vi "gyro pll async.vi"(11 "pll event pair":T8) -> ()   [LabVIEW 2018]
uses:
  agregator -- action.ctl
  four-corner circle transformation.ctl
  interpolation state - real.ctl
  PID action.ctl
  data source action.ctl
  publisher action.ctl
  pll talkback data type.ctl
  server talkback message type.ctl
  pid -- parameters.ctl
  PID - mode.ctl
  pll parameters.ctl
  lorentzian.ctl
  circle corners.ctl
  server talkto message type.ctl
  server talk-to-back pair.ctl
panel:
  in  "main":enum32{"Page 1", "Page 2", "Page 3"}(tab)
  in  "pll parameters":T1={"PID mode"=enum."normal", "plot hist time (sec)"=1.0, "dt (sec)"=0.001, "visc hist time (sec)"=2.0, "time int ave time (sec)"=0.3, "PLL limits (Hz)"=5000.0} {"PLL limits (Hz)" format="%#.2f"; "time int ave time (sec)" format="%#_10f"; "visc hist time (sec)" format="%#_10f"; "dt (sec)" format="%#_10f"; "plot hist time (sec)" format="%#_10f"}
  in  "PID parameters :{}[];'":T3={"I (sec)"=0.004634123928756344, "P (sec)"=0.008980860327047186} {"P (sec)" scale=0.01..10.0; "I (sec)" scale=0.01..10.0}
  out "results":T4={"freq (Hz)"=40017.438097734725, "gamma (Hz)"=6.817921124952451, "Voltage (V)"=6.817921124952451+0.0i, "overlimit ?"=FALSE} {"Voltage (V)" format="%#.4f"; "gamma (Hz)" format="%#.4f"; "freq (Hz)" format="%#.11f"}
  out "PLL is ON ?":bool
  in  "Do reset frequency -- PID action":T5=enum."reset frequency"
  in  "Do reset frequency source":dbl=15.0 format="%#_10f"
  out "zi freq temporary":dbl=40015.59220124337 format="%#.2f"
  out "DO reset freq !":bool
  in  "lorentzian":T6={"A (VHz)"=1.0, "f (Hz)"=1000.0, "G (Hz)"=3.0, "phi(rad)"=0.0, "Q"=300.0, "Norm  Ampl"=nan, "bg (V)"=0.0+0.0i, "4corners"={"z (-pi/2)"=9.277908004825974e-07+0.0007240755403629966i, "z(inf)"=2.6527949823343002e-05+0.0007477540585896028i, "z (pi/2)"=2.8494315967368497e-06+0.0007733542176124632i, "z center"=1.8886111986097237e-06+0.0007487148789877299i, "z(0)"=-2.2750727426123552e-05+0.000749675699385857i, "radius"=2.4658065287076567e-05}} {"bg (V)" format="%#9_9f"; "Q" format="%#9_9f"; "phi(rad)" format="%#9_9f"; "G (Hz)" format="%#9_9f"; "f (Hz)" format="%#9_9f"}
  out "Stoped?":bool
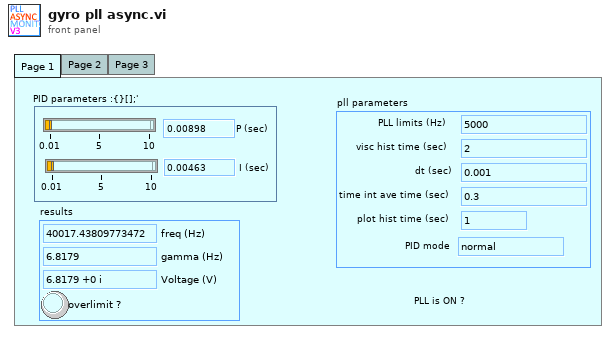
[diagram p1: front panel]
types:
  T1 = typedef "pll parameters.ctl" = cluster{"PID mode":T2, "plot hist time (sec)":dbl, "dt (sec)":dbl, "visc hist time (sec)":dbl, "time int ave time (sec)":dbl, "PLL limits (Hz)":dbl}
  T2 = typedef "PID - mode.ctl" = enum16{"normal", "heat"}
  T3 = typedef "pid -- parameters.ctl" = cluster{"I (sec)":dbl, "P (sec)":dbl}
  T4 = typedef "pll talkback data type.ctl" = cluster{"freq (Hz)":dbl, "gamma (Hz)":dbl, "Voltage (V)":cdb, "overlimit ?":bool}
  T5 = typedef "PID action.ctl" = enum16{"append", "empty!", "reset frequency", "reset from num", "overlimit"}
  T6 = typedef "lorentzian.ctl" = cluster{"A (VHz)":dbl, "f (Hz)":dbl, "G (Hz)":dbl, "phi(rad)":dbl, "Q":dbl, "Norm  Ampl":dbl, "bg (V)":cdb, "4corners":T7}
  T7 = typedef "circle corners.ctl" = cluster{"z (-pi/2)":cdb, "z(inf)":cdb, "z (pi/2)":cdb, "z center":cdb, "z(0)":cdb, "radius":dbl}
  T8 = typedef "server talk-to-back pair.ctl" = cluster{"talkback event":refnum<user-event>, "talkto event":refnum<user-event>}
  T9 = typedef "interpolation state - real.ctl" = cluster{"requested size":i32, "Array":dbl[], "actual number of elements":i32}
  T10 = typedef "agregator -- action.ctl" = enum16{"append", "interpolate", "empty!", "force", "init", "scale", "read last"}
  T11 = typedef "server talkback message type.ctl" = cluster{"message":enum16{"new", "void"}}
  T12 = typedef "publisher action.ctl" = enum16{"set", "get", "init", "check"}
  T13 = typedef "data source action.ctl" = enum16{"set", "get", "init", "set-and-get", "init source"}
  T14 = typedef "four-corner circle transformation.ctl" = enum16{"z(c) z(inf)", "z(c) z(zero)", "fix phase", "calculate lorentzian", "z(0) z(+-pi/2)", "shift to zcenter", "to  canonical", "get canonical phase", "get4corners", "update lorentzian -- from z0", "fake gamma normal", "fake gamma heat", "calculate complex slope"}
  T15 = typedef "PLL data source.ctl" = enum16{"meta", "MFLI", "SRS865A", "arydh"}
  T16 = typedef "interpolation state - complex.ctl" = cluster{"requested size":i32, "Array":cdb[], "actual number of elements":i32}
  T17 = enum16{"stop", "start", "update pars", "update request", "new", "launch", "exit", "get", "reset", "pause", "unpause"}
  T18 = typedef "eventvkey.ctl" = enum16{"ASCII", "Enter", "Return", "Shift", "Ctrl", "Alt", "Cmd", "Opt", "Caps", "NumLock", "Clear", "Break", "Up", "Down", "Left", "Right", "Insert", "Delete", "Home", "End", "PageUp", "PageDown", "Escape", "Help", "Pause", "ScrollLock", "F1", "F2", "F3", "F4", "F5", "F6", "F7", "F8", "F9", "F10", "F11", "F12", "F13", "F14", "F15", "F16", "F17", "F18", "F19", "F20", "F21", "F22", "F23", "F24", "Play", "VolumeUp", "VolumeDown", "Mute", "Two Byte Char"}
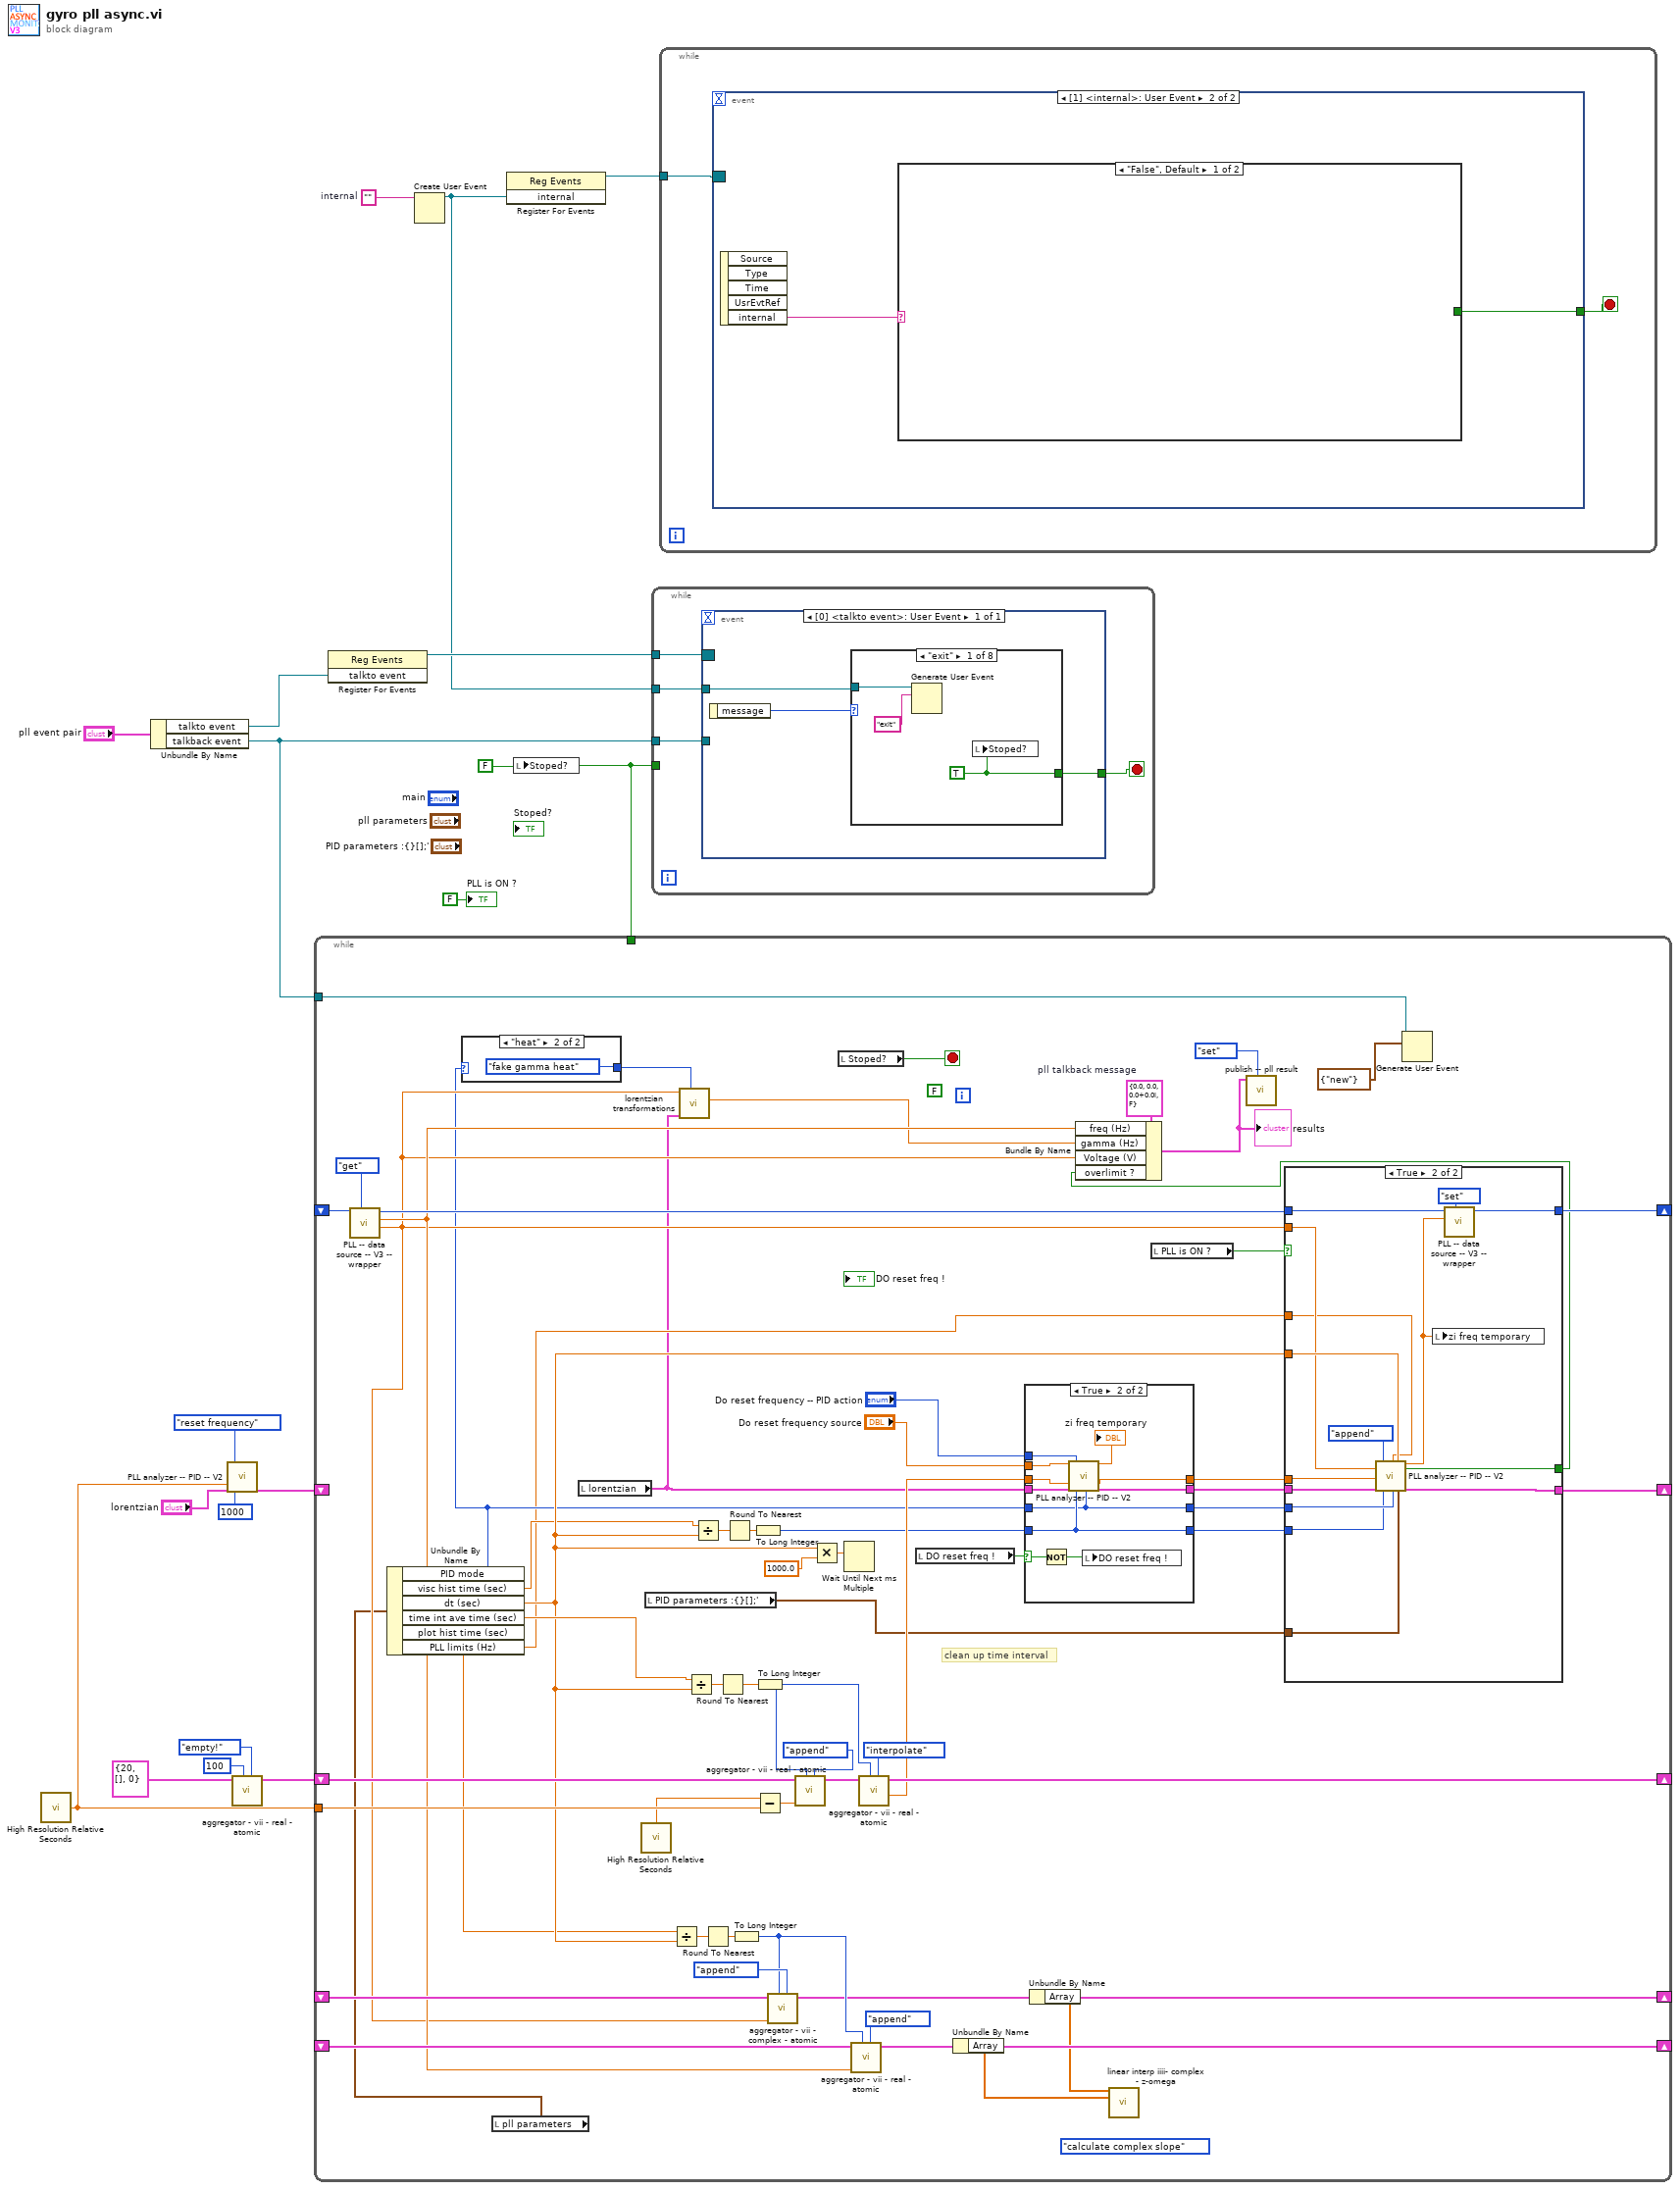
[diagram p0: block diagram]
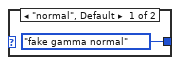
[diagram p2: hidden frame]
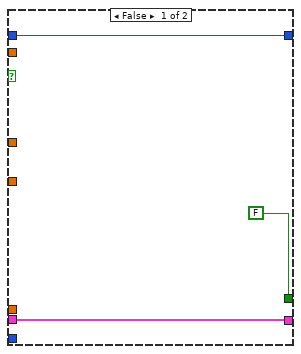
[diagram p3: hidden frame]
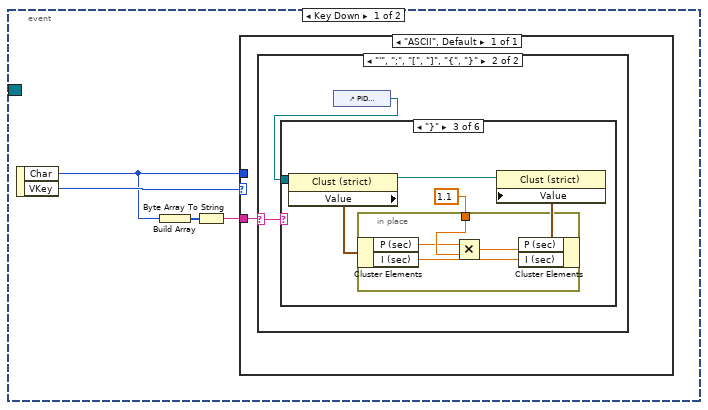
[diagram p5: hidden frame]
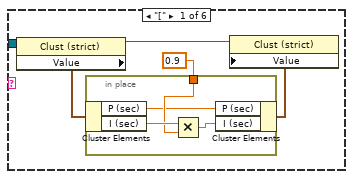
[diagram p7: hidden frame]
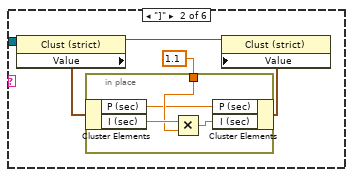
[diagram p8: hidden frame]
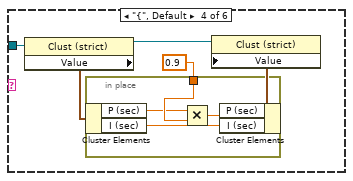
[diagram p9: hidden frame]
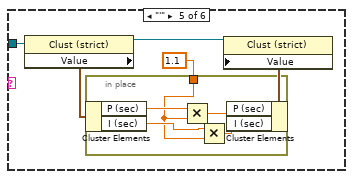
[diagram p10: hidden frame]
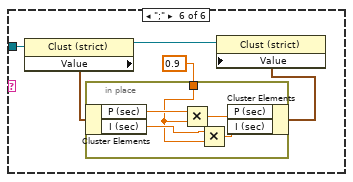
[diagram p11: hidden frame]
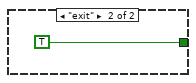
[diagram p12: hidden frame]
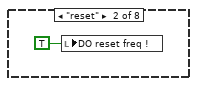
[diagram p13: hidden frame]
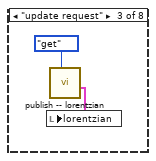
[diagram p14: hidden frame]
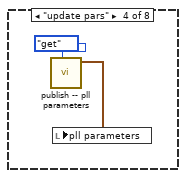
[diagram p15: hidden frame]
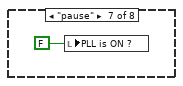
[diagram p18: hidden frame]
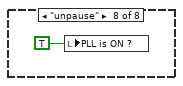
[diagram p19: hidden frame]
diagram:
  w3 = ""  # internal
  w4 = FALSE ("Stop")
  n1 = call <vilib>:"High Resolution Relative Seconds.vi"() -> ("relative seconds"=w6:dbl)
  n2 = Unbundle By Name("pll event pair") -> ("talkto event"=w14:refnum<user-event>, "talkback event"=w15:refnum<user-event>)
  n3 = call "PLL analyzer -- PID -- V2.vi"("time in (sec)"=w6, "lorentzian IN"="lorentzian", "PID action"=PID_action."reset frequency", "requested size"=1000) -> ("lorentzian  OUT"=w9:T6)  [unwired: 12 in, 3 out]
  n4 = call "aggregator - vii - real - atomic.vi"("aggregator action"=agregator_--_action."empty!", "requested size"=100, "state IN"=T9 {"requested size"=20, "Array"=[], "actual number of elements"=0}) -> ("state OUT"=w12:T9)  [unwired: 5 in, 3 out]
  n5 = while {
    tunnel: w6 -> [w79]
    shift-right: [w77] -> _
    shift-left: w9 -> [_]
    shift-right: [w43] -> _
    shift-left: _ -> [w76]
    shift-right: [w72] -> _
    shift-left: _ -> [w73]
    shift-right: [w67] -> _
    shift-left: w12 -> [w70]
    shift-right: [w62] -> _
    shift-left: _ -> [w58]
    tunnel: w15 -> [w20]
    tunnel: w4 -> [_]
    stop <- w23 stop-if-true
    (unwired) FALSE
    w35 = T4 {"freq (Hz)"=0.0, "gamma (Hz)"=0.0, "Voltage (V)"=0.0+0.0i, "overlimit ?"=FALSE}  # pll talkback message
    (unwired) four-corner_circle_transformation."calculate complex slope" ("4 corner circle transformation")
    # "clean up time interval"
    n6 = call "PLL -- data source -- V3 -- wrapper.vi"("data source action"=data_source_action."get", "PLL data source"=w58) -> ("z out (V)"=w38:cdb, "Freq out (Hz)"=w42:dbl, "PLL data source OUT"=w60:T15)  [unwired: 7 in]
    n7 = local read "pll parameters"() -> (w30:T1)
    n8 = Unbundle By Name(w30) -> ("PID mode"=w31:T2, "visc hist time (sec)"=w32:dbl, "dt (sec)"=w33:dbl, "time int ave time (sec)"=w34:dbl, "plot hist time (sec)"=w29:dbl, "PLL limits (Hz)"=w27:dbl)
    n9 = case shown="\"heat\"" w31 {
      tunnel: [four-corner_circle_transformation."fake gamma normal" ("4 corner circle transformation") four-corner_circle_transformation."fake gamma heat" ("4 corner circle transformation")] -> w40
      frame "normal", Default {
      }
      frame "heat" {
      }
    }
    n10 = local read "lorentzian"() -> (w24:T6)
    n11 = call <vilib>:"High Resolution Relative Seconds.vi"() -> ("relative seconds"=w61:dbl)
    n12 = local read "PID parameters :{}[];'"() -> (w21:T3)
    n13 = Divide(x=w29, y=w33) -> (x/y=w47:dbl)
    n14 = call "lorentzian transformations.vi"("4 corner circle transformation"=w40, "lorentzian in"=w24, "voltage in"=w38) -> ("gamma OUT"=w39:dbl)  [unwired: 5 in, 3 out]
    n15 = Divide(x=w34, y=w33) -> (x/y=w51:dbl)
    n16 = Divide(x=w32, y=w33) -> (x/y=w54:dbl)
    n17 = Round To Nearest(number=w47) -> (nearest integer value=w46:dbl)
    n18 = Round To Nearest(number=w51) -> (nearest integer value=w50:dbl)
    n19 = Round To Nearest(number=w54) -> (nearest integer value=w53:dbl)
    n20 = To Long Integer(number=w46) -> (32bit integer=w45:i32)
    n21 = To Long Integer(number=w53) -> (32bit integer=w52:i32)
    n22 = To Long Integer(number=w50) -> (32bit integer=w49:i32)
    n23 = Subtract(x=w61, y=w79) -> (x-y=w69:dbl)
    n24 = call "aggregator - vii - complex - atomic.vi"("aggregator action"=agregator_--_action."append", "requested size"=w45, "number"=w38, "state IN"=w76) -> ("state OUT"=w43:T16)  [unwired: 4 in, 3 out]
    n25 = call "aggregator - vii - real - atomic.vi"("aggregator action"=agregator_--_action."append", "requested size"=w49, "number"=w69, "state IN"=w70) -> ("state OUT"=w68:T9)  [unwired: 4 in, 3 out]
    n26 = Multiply(x=w33, y=1000.0) -> (x*y=w65:dbl)
    n27 = local read "Stoped?"() -> (w23:bool)
    n28 = Wait Until Next ms Multiple(millisecond multiple=w65) -> ()  [unwired: 1 out]
    n29 = call "aggregator - vii - real - atomic.vi"("aggregator action"=agregator_--_action."append", "requested size"=w45, "number"=w42, "state IN"=w73) -> ("state OUT"=w72:T9)  [unwired: 4 in, 3 out]
    n30 = call "aggregator - vii - real - atomic.vi"("aggregator action"=agregator_--_action."interpolate", "requested size"=w49, "state IN"=w68) -> ("interp average"=w56:dbl, "state OUT"=w67:T9)  [unwired: 5 in, 2 out]
    n31 = local read "DO reset freq !"() -> (w64:bool)
    n32 = Unbundle By Name(w72) -> ("Array"=w36:dbl[])
    n33 = case shown="True" w64 {
      selector: w64 -> [_ w112]
      tunnel: w24 -> [w103 w114]
      tunnel: [w103 w113] -> w63
      tunnel: w52 -> [w102 w109]
      tunnel: [w102 w109] -> w57
      tunnel: w56 -> [w101 w108]
      tunnel: "Do reset frequency -- PID action" -> [_ w107]
      tunnel: "Do reset frequency source" -> [_ w106]
      tunnel: [w101 w105] -> w48
      tunnel: w31 -> [w100 w104]
      tunnel: [w100 w104] -> w44
      frame False {
      }
      frame True {
        n34 = Not(x=w112) -> (.not. x?=w111:bool)
        n35 = call "PLL analyzer -- PID -- V2.vi"("frequency IN (Hz)"=w106, "time in (sec)"=w108, "lorentzian IN"=w114, "PID action"=w107, "requested size"=w109, "PID mode"=w104) -> ("frequency OUT (Hz)"=→"zi freq temporary":dbl, "time out (sec)"=w105:dbl, "lorentzian  OUT"=w113:T6)  [unwired: 10 in, 1 out]
        n36 = local write "DO reset freq !"(w111) -> ()
      }
    }
    n37 = Unbundle By Name(w43) -> ("Array"=w37:cdb[])
    n38 = call "linear interp iiii- complex - z-omega.vi"("z"=w37, "omega"=w36) -> ()  [unwired: 5 in, 9 out]
    n39 = local read "PLL is ON ?"() -> (w22:bool)
    n40 = case shown="True" w22 {
      tunnel: [w84 w99] -> w77
      tunnel: w57 -> [_ w90]
      tunnel: w38 -> [_ w88]
      tunnel: w48 -> [_ w94]
      tunnel: w63 -> [w84 w91]
      tunnel: [w83 w97] -> w62
      tunnel: w60 -> [w83 w95]
      tunnel: w33 -> [_ w93]
      tunnel: w44 -> [_ w92]
      tunnel: w21 -> [_ w87]
      tunnel: [FALSE w86] -> w28
      tunnel: w27 -> [_ w85]
      frame False {
      }
      frame True {
        n41 = call "PLL analyzer -- PID -- V2.vi"("voltage IN (V)"=w88, "time in (sec)"=w94, "lorentzian IN"=w91, "PID action"=PID_action."append", "requested size"=w90, "PLL limits (Hz)"=w85, "PID mode"=w92, "dt (sec)"=w93, "PID parameters"=w87) -> ("frequency OUT (Hz)"=w89:dbl, "overlimit ?"=w86:bool, "lorentzian  OUT"=w99:T6)  [unwired: 7 in, 1 out]
        n42 = local write "zi freq temporary"(w89) -> ()
        n43 = call "PLL -- data source -- V3 -- wrapper.vi"("data source action"=data_source_action."set", "Freq in (Hz)"=w89, "PLL data source"=w95) -> ("PLL data source OUT"=w97:T15)  [unwired: 6 in, 2 out]
      }
    }
    n44 = Bundle By Name(cluster=w35, "freq (Hz)"=w42, "gamma (Hz)"=w39, "Voltage (V)"=w38, "overlimit ?"=w28) -> (w26:T4)
    "results" <- w26
    n45 = call "publish -- pll result.vi"("publisher action"=publisher_action."set", "pll result IN"=w26) -> ()  [unwired: 9 in, 1 out]
    n46 = Generate User Event(user event=w20, event data cluster=T11 {"message"=enum."new"} ("event data")) -> ()  [unwired: 2 in, 2 out]
  }
  n47 = register-events(w14) -> (reference out=w18:refnum<event-registration>)  [unwired: 2 in, 1 out]
  n48 = Create User Event(user event datatype=w3) -> (user event=w1:refnum<user-event>)  [unwired: 1 in, 1 out]
  n49 = register-events(w1) -> (reference out=w2:refnum<event-registration>)  [unwired: 2 in, 1 out]
  n50 = local write "Stoped?"(w4) -> ()
  n51 = while {
    tunnel: w18 -> [w118]
    tunnel: w15 -> [w117]
    tunnel: w4 -> [_]
    tunnel: w1 -> [w115]
    stop <- w116 stop-if-true
    n52 = event shown="[0] <talkto event>: User Event" {
      selector: w118 -> [_]
      dyn-events: _ -> [_]
      timeout: _ -> [_]
      tunnel: w117 -> [_]
      tunnel: [w120] -> w116
      tunnel: w115 -> [w119]
      event User Event {
        n53 = event-data() -> ("message"=w121:T17)  [unwired: 1 in]
        n54 = case shown="\"exit\"" w121 {
          tunnel: [w124 _ _ _ _ _ _ _] -> w120
          tunnel: w119 -> [w123 _ _ _ _ _ _ _]
          frame "exit" {
            w124 = TRUE
            n55 = Generate User Event(user event=w123, event data cluster="exit" ("event data")) -> ()  [unwired: 2 in, 2 out]
            n56 = local write "Stoped?"(w124) -> ()
          }
          frame "reset" {
            n57 = local write "DO reset freq !"(TRUE) -> ()
          }
          frame "update request" {
            n58 = call "publish -- lorentzian.vi"("publisher action"=publisher_action."get") -> ("lorentzian OUT"=w126:T6)  [unwired: 10 in]
            n59 = local write "lorentzian"(w126) -> ()
          }
          frame "update pars" {
            n60 = call "publish -- pll parameters.vi"("publisher action"=publisher_action."get") -> ("pll parameters OUT"=w128:T1)  [unwired: 10 in]
            n61 = local write "pll parameters"(w128) -> ()
          }
          frame "start", Default {
          }
          frame "stop" {
          }
          frame "pause" {
            n62 = local write "PLL is ON ?"(FALSE ("Stoped?")) -> ()
          }
          frame "unpause" {
            n63 = local write "PLL is ON ?"(TRUE ("Stoped?")) -> ()
          }
        }
      }
    }
  }
  n64 = while {
    tunnel: w2 -> [w133]
    stop <- w132 stop-if-true
    n65 = event shown="[1] <internal>: User Event" {
      selector: w133 -> [_ _]
      dyn-events: _ -> [_ _]
      timeout: _ -> [_ _]
      tunnel: [_ w197] -> w132
      event Key Down {
        n66 = event-data() -> ("Char"=w135:i16, "VKey"=w137:T18)  [unwired: 1 in]
        n67 = Build Array(w135) -> (w136:i16[])
        n68 = Byte Array To String(unsigned byte array=w136) -> (string=w134:string)
        n69 = case shown="\"ASCII\", Default" w137 {
          tunnel: w135 -> [_]
          tunnel: w134 -> [w138]
          frame "ASCII", Default {
            n70 = case shown="\"'\", \";\", \"[\", \"]\", \"{\", \"}\"" w138 {
              selector: w138 -> [_ w140]
              frame "0", Default {
              }
              frame "'", ";", "[", "]", "{", "}" {
                n71 = control-ref of="PID parameters :{}[];'"() -> (w139:refnum<vi>)
                n72 = case shown="\"}\"" w140 {
                  tunnel: w139 -> [w145 w154 w163 w172 w181 w191]
                  frame "[" {
                    n73 = property class="Clust (strict)"(reference=w145) -> (reference out=w144:refnum<vi>, "Value"=w143:T3)  [unwired: 1 in, 1 out]
                    n74 = in-place {
                      in-place-border: 0.9 -> [w148]
                      n75 = in-place-cluster #1(w143) -> ("P (sec)"=w146:dbl, "I (sec)"=w149:dbl)
                      n76 = Multiply(x=w149, y=w148) -> (x*y=w147:dbl)
                      n77 = in-place-cluster #1("P (sec)"=w146, "I (sec)"=w147) -> (w142:T3)
                    }
                    n78 = property class="Clust (strict)"(reference=w144, "Value"=w142) -> ()  [unwired: 1 in, 2 out]
                  }
                  frame "]" {
                    n79 = property class="Clust (strict)"(reference=w154) -> (reference out=w153:refnum<vi>, "Value"=w152:T3)  [unwired: 1 in, 1 out]
                    n80 = in-place {
                      in-place-border: 1.1 -> [w157]
                      n81 = in-place-cluster #2(w152) -> ("P (sec)"=w155:dbl, "I (sec)"=w158:dbl)
                      n82 = Multiply(x=w158, y=w157) -> (x*y=w156:dbl)
                      n83 = in-place-cluster #2("P (sec)"=w155, "I (sec)"=w156) -> (w151:T3)
                    }
                    n84 = property class="Clust (strict)"(reference=w153, "Value"=w151) -> ()  [unwired: 1 in, 2 out]
                  }
                  frame "}" {
                    n85 = property class="Clust (strict)"(reference=w163) -> (reference out=w162:refnum<vi>, "Value"=w161:T3)  [unwired: 1 in, 1 out]
                    n86 = in-place {
                      in-place-border: 1.1 -> [w167]
                      n87 = in-place-cluster #3(w161) -> ("P (sec)"=w166:dbl, "I (sec)"=w164:dbl)
                      n88 = Multiply(x=w166, y=w167) -> (x*y=w165:dbl)
                      n89 = in-place-cluster #3("P (sec)"=w165, "I (sec)"=w164) -> (w160:T3)
                    }
                    n90 = property class="Clust (strict)"(reference=w162, "Value"=w160) -> ()  [unwired: 1 in, 2 out]
                  }
                  frame "{", Default {
                    n91 = property class="Clust (strict)"(reference=w172) -> (reference out=w171:refnum<vi>, "Value"=w170:T3)  [unwired: 1 in, 1 out]
                    n92 = in-place {
                      in-place-border: 0.9 -> [w176]
                      n93 = in-place-cluster #4(w170) -> ("P (sec)"=w175:dbl, "I (sec)"=w173:dbl)
                      n94 = Multiply(x=w175, y=w176) -> (x*y=w174:dbl)
                      n95 = in-place-cluster #4("P (sec)"=w174, "I (sec)"=w173) -> (w169:T3)
                    }
                    n96 = property class="Clust (strict)"(reference=w171, "Value"=w169) -> ()  [unwired: 1 in, 2 out]
                  }
                  frame "'" {
                    n97 = property class="Clust (strict)"(reference=w181) -> (reference out=w180:refnum<vi>, "Value"=w179:T3)  [unwired: 1 in, 1 out]
                    n98 = in-place {
                      in-place-border: 1.1 -> [w182]
                      n99 = in-place-cluster #5(w179) -> ("P (sec)"=w186:dbl, "I (sec)"=w184:dbl)
                      n100 = Multiply(x=w186, y=w182) -> (x*y=w185:dbl)
                      n101 = Multiply(x=w184, y=w182) -> (x*y=w183:dbl)
                      n102 = in-place-cluster #5("P (sec)"=w185, "I (sec)"=w183) -> (w178:T3)
                    }
                    n103 = property class="Clust (strict)"(reference=w180, "Value"=w178) -> ()  [unwired: 1 in, 2 out]
                  }
                  frame ";" {
                    n104 = property class="Clust (strict)"(reference=w191) -> (reference out=w190:refnum<vi>, "Value"=w189:T3)  [unwired: 1 in, 1 out]
                    n105 = in-place {
                      in-place-border: 0.9 -> [w192]
                      n106 = in-place-cluster #6(w189) -> ("P (sec)"=w196:dbl, "I (sec)"=w194:dbl)
                      n107 = Multiply(x=w196, y=w192) -> (x*y=w195:dbl)
                      n108 = Multiply(x=w194, y=w192) -> (x*y=w193:dbl)
                      n109 = in-place-cluster #6("P (sec)"=w195, "I (sec)"=w193) -> (w188:T3)
                    }
                    n110 = property class="Clust (strict)"(reference=w190, "Value"=w188) -> ()  [unwired: 1 in, 2 out]
                  }
                }
              }
            }
          }
        }
      }
      event User Event {
        n111 = event-data() -> ("internal"=w198:string)  [unwired: 1 in, 4 out]
        n112 = case shown="\"False\", Default" w198 {
          tunnel: [_ TRUE] -> w197
          frame "False", Default {
          }
          frame "exit" {
          }
        }
      }
    }
  }
  "PLL is ON ?" <- FALSE ("unpaused?")
